vi "Execute.vi"(8 "error in":errorcluster, 11 "O2 Flow Rate STEP in":refnum<class "Pressure Control Rate STEP.lvclass">) -> (0 "error out":errorcluster, 1 "Next Step?":bool, 2 "MSG":string, 3 "O2 Flow Rate STEP out":refnum<class "Pressure Control Rate STEP.lvclass">)   [LabVIEW 2014, in "Pressure Control Rate STEP.lvclass"]
uses:
  Pressure Control Rate STEP.lvclass
  <vilib>/ActorFramework/Message Enqueuer/Message Enqueuer.lvclass
  Controller/Messages/Update Device Setpoint MSG/Update Device Setpoint.lvclass
  reusable/Sequence/STEPS/STEP.lvclass/STEP.ctl
  reusable/Sequence/STEPS/LEAVES/Double/Switch DBL.lvclass/Switch DBL.ctl
  Controller/Messages/Update Device Setpoint MSG/Update Device Setpoint.lvclass/Update Device Setpoint.ctl
  <vilib>/ActorFramework/Message Enqueuer/Message Enqueuer.lvclass/Message Enqueuer.ctl
  reusable/Sequence/STEPS/Read Obj.vi
  reusable/Sequence/STEPS/LEAVES/Double/Read val.vi
  Controller/Messages/Update Device Setpoint MSG/Write SP.vi
  Controller/Messages/Update Device Setpoint MSG/Write DevID.vi
  <vilib>/ActorFramework/Message Priority Queue/Priority Enqueue.vi
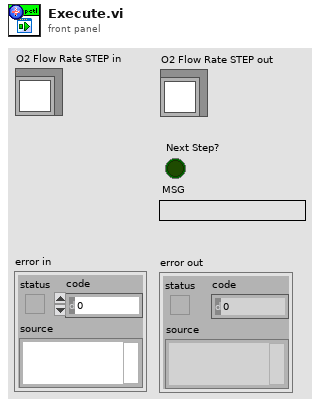
[diagram p1: front panel]
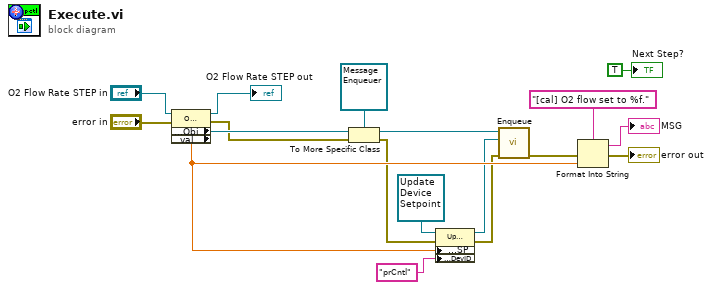
[diagram p0: block diagram]
diagram:
  n1 = property class="O2 Flow Rate"(reference="O2 Flow Rate STEP in", error in="error in") -> (reference out=→"O2 Flow Rate STEP out":refnum<class "Pressure Control Rate STEP.lvclass">, error out=w16:errorcluster, "Accessors:Obj"=w18:refnum<class>, "val"=w7:dbl)
  n2 = To More Specific Class(target class=refnum<class "Message Enqueuer.lvclass"> refnum ("Message Enqueuer in"), reference=w18, error in=w16) -> (specific class reference=w15:refnum<class "Message Enqueuer.lvclass">, error out=w5:errorcluster)
  n3 = property class="Update Device Setpoint"(reference=refnum<class "Update Device Setpoint.lvclass"> refnum ("Controller:Update Device Setpoint"), error in=w5, "Accessors:SP"=w7, "Accessors:DevID"="prCntl" ("DevID")) -> (reference out=w6:refnum<class "Update Device Setpoint.lvclass">, error out=w4:errorcluster)
  n4 = call <vilib>:"Enqueue.vi"("error in (no error)"=w4, "Message"=w6, "Message Enqueuer in"=w15) -> ("error out"=w13:errorcluster)  [unwired: 7 in, 1 out]
  n5 = Format Into String(format string="[cal] O2 flow set to %f.", error in=w13, w7) -> (resulting string=→"MSG":string, error out=→"error out":errorcluster)  [unwired: 1 in]
  "Next Step?" <- TRUE ("Next Step?")
